vi "CDMA_RxFrameSyn.vi"(7 "timeslot_star":dbl, 8 "error in (no error)":errorcluster caption="错误输入（无错误）", 9 "sampleRate":dbl, 10 "rx_data":cdb[](array[numeric]), 11 "Path In":path) -> (0 "error out":errorcluster caption="错误输出", 1 "scrambleGroupNo":dbl, 2 "searchFlag1":dbl, 3 "Path Out":path, 4 "rx_data1":cdb[](array[numeric]), 5 "firstTimeslotNo":dbl)   [LabVIEW 2015]
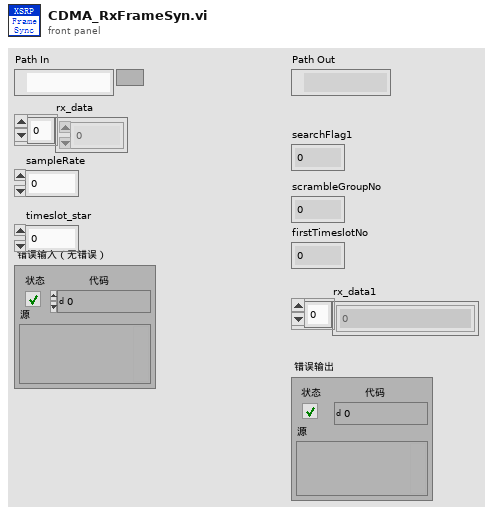
[diagram p1: front panel]
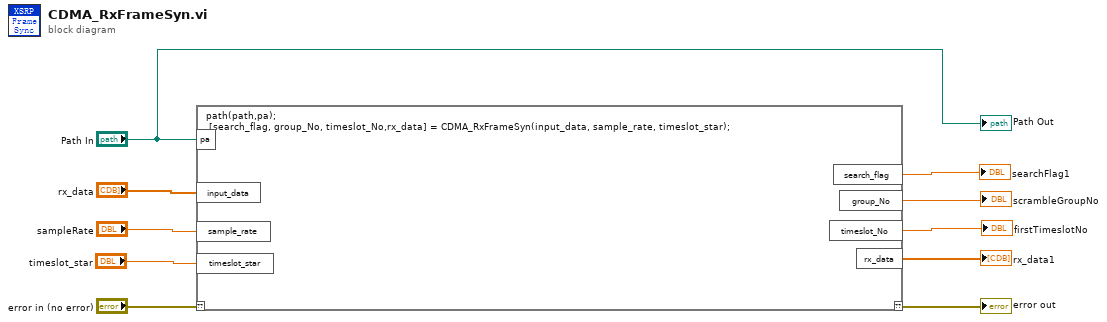
[diagram p0: block diagram]
diagram:
  n1 = script code="path(path,pa);\n [search_flag, group_No, timeslot_No,rx_data] = CDMA_RxFrameSyn(input_data, sample_rate, timeslot_star);"("??"="error in (no error)", "pa"="Path In", "input_data"="rx_data", "sample_rate"="sampleRate", "timeslot_star"="timeslot_star") -> ("??"=→"error out":errorcluster, "search_flag"=→"searchFlag1":dbl, "group_No"=→"scrambleGroupNo":dbl, "timeslot_No"=→"firstTimeslotNo":dbl, "rx_data"=→"rx_data1":cdb[])
  "Path Out" <- "Path In"
